vi "Timeout during execution--error.vi"() -> (0 "error out":errorcluster)   [LabVIEW 2025]
doc: "Indicates that the executed process did not terminate within the configured timeout period. This error is raised when a finite timeout is specified and the process fails to complete in time."
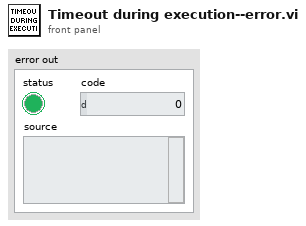
[diagram p1: front panel]
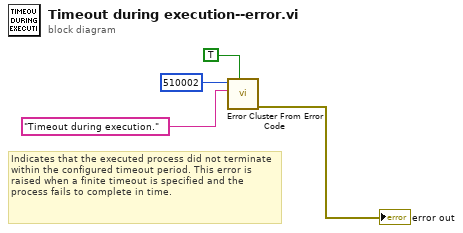
[diagram p0: block diagram]
diagram:
  # "Indicates that the executed process did not terminate within the configured timeout period. This error is raised when a finite timeout is specified and the process fails to complete in time."
  n1 = call <vilib>:"Error Cluster From Error Code.vi"("show call chain? (False)"=TRUE, "error message (\"\")"="Timeout during execution." ("error message (\"\")"), "error code (0)"=510002) -> ("error out"=→"error out":errorcluster)  [unwired: 6 in]
